vi "Split the Work.vi"(11 "Volcano":refnum<class "Volcano.lvclass">) -> (2 "Elephant's Volcanoes":refnum<class "Volcano.lvclass">[](array[class]), 3 "My Volcanoes":refnum<class "Volcano.lvclass">[](array[class]))   [LabVIEW 2023, in "d16.lvlib" / "Volcano.lvclass"]
uses:
  Volcano.lvclass
  Volcano.lvclass/Volcano.ctl
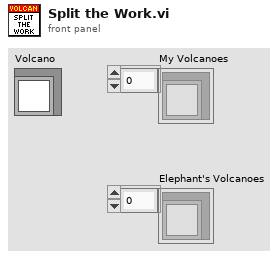
[diagram p1: front panel]
types:
  T1 = cluster{"Current Valve":string, "Unopened Valves":string[], "Cumulative Pressure Released":u64, "Time":i32}[]
  T2 = cluster{"Current Valve":string, "Unopened Valves":string[], "Cumulative Pressure Released":u64, "Time":i32}
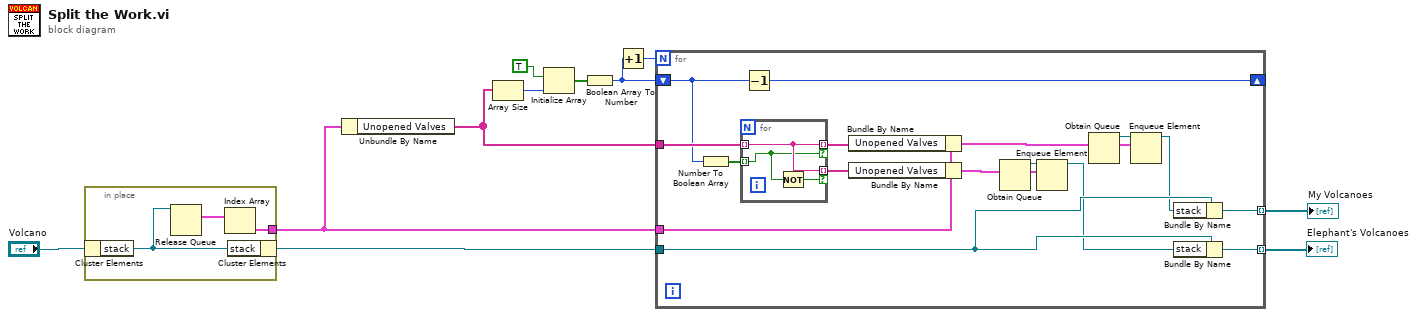
[diagram p0: block diagram]
diagram:
  n1 = in-place {
    in-place-border: [w12] -> w4
    n2 = in-place-cluster #1("Volcano") -> ("stack"=w14:refnum<queue>)
    n3 = Release Queue(queue=w14) -> (remaining elements=w13:T1)  [unwired: 2 in, 2 out]
    n4 = Index Array(array=w13) -> (element=w12:T2)  [unwired: 1 in]
    n5 = in-place-cluster #1("stack"=w14) -> (w3:refnum<class "Volcano.lvclass">)
  }
  n6 = Unbundle By Name(w4) -> ("Unopened Valves"=w8:string[])
  n7 = Array Size(array=w8) -> (size(s)=w7:i32)
  n8 = Initialize Array(TRUE, w7) -> (w9:bool[])
  n9 = Boolean Array To Number(Boolean array=w9) -> (number=w6:u32)
  n10 = Increment(x=w6) -> (x+1=w5:u32)
  n11 = for {
    N: w5 -> [_]
    shift-right: [w30] -> _
    shift-left: w6 -> [w28]
    tunnel: w8 -> [w29]
    tunnel: w4 -> [w24]
    tunnel: w3 -> [w22]
    tunnel: [w20] -> w2 mode=indexing
    tunnel: [w19] -> w1 mode=indexing
    n12 = Number To Boolean Array(number=w28) -> (Boolean array=w27:bool[])
    n13 = for {
      tunnel: w29 -> [w33] mode=indexing
      tunnel: w27 -> [w32] mode=indexing
      tunnel: [w33] -> w25 mode=indexing if=w32
      tunnel: [w33] -> w26 mode=indexing if=w31
      n14 = Not(x=w32) -> (.not. x?=w31:bool)
    }
    n15 = Decrement(x=w28) -> (x-1=w30:u32)
    n16 = Bundle By Name(cluster=w24, "Unopened Valves"=w25) -> (w21:T2)
    n17 = Bundle By Name(cluster=w24, "Unopened Valves"=w26) -> (w23:T2)
    n18 = Obtain Queue(element data type=w23) -> (queue out=w18:refnum<queue>)  [unwired: 4 in, 2 out]
    n19 = Enqueue Element(queue=w18, element=w23) -> (queue out=w16:refnum<queue>)  [unwired: 2 in, 2 out]
    n20 = Obtain Queue(element data type=w21) -> (queue out=w17:refnum<queue>)  [unwired: 4 in, 2 out]
    n21 = Enqueue Element(queue=w17, element=w21) -> (queue out=w15:refnum<queue>)  [unwired: 2 in, 2 out]
    n22 = Bundle By Name(cluster=w22, "stack"=w15) -> (w20:refnum<class "Volcano.lvclass">)
    n23 = Bundle By Name(cluster=w22, "stack"=w16) -> (w19:refnum<class "Volcano.lvclass">)
  }
  "My Volcanoes" <- w2
  "Elephant's Volcanoes" <- w1
